vi "外设配置对话框.vi"() -> ()   [LabVIEW 2016, in "斯坦道CODCr.lvlib"]
uses:
  <vilib>/Utility/miscctls.llb/LVPointTypeDef.ctl
panel:
  in  "外设配置":T1 {"总氮x公式0" items=["0", "1"]; "光谱仪类型" items=["1型", "2型", "3型", "2型氙灯联控"]; "泵阀量" items=["9通"=9, "10通"=10, "12通"=12]; "泵类型" items=["1型", "2型", "sy04型+旋转阀"]}
  in  "关闭":bool
  in  "保存":bool
  in  "读取":bool
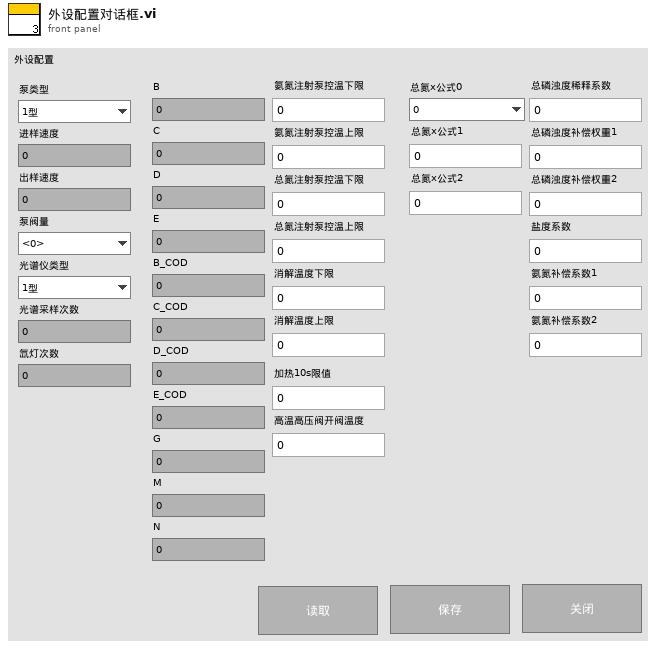
[diagram p1: front panel]
types:
  T1 = cluster{"泵类型":u8, "进样速度":u32, "出样速度":u32, "泵阀量":u8, "光谱仪类型":u8, "光谱采样次数":u8, "氙灯次数":u8, "B":u16, "C":u16, "D":u16, "E":u16, "B_COD":u16, "C_COD":u16, "D_COD":u16, "E_COD":u16, "G":u16, "M":u16, "N":u16, "氨氮注射泵控温下限":sgl, "氨氮注射泵控温上限":sgl, "总氮注射泵控温下限":sgl, "总氮注射泵控温上限":sgl, "消解温度下限":sgl, "消解温度上限":sgl, "加热10s限值":sgl, "高温高压阀开阀温度":sgl, "总氮x公式0":u8, "总氮x公式1":sgl, "总氮x公式2":sgl, "总磷浊度稀释系数":sgl, "总磷浊度补偿权重1":sgl, "总磷浊度补偿权重2":sgl, "盐度系数":sgl, "氨氮补偿系数1":sgl, "氨氮补偿系数2":sgl}
  T2 = typedef "LVPointTypeDef.ctl" = cluster{"Horizontal":i16, "Vertical":i16}
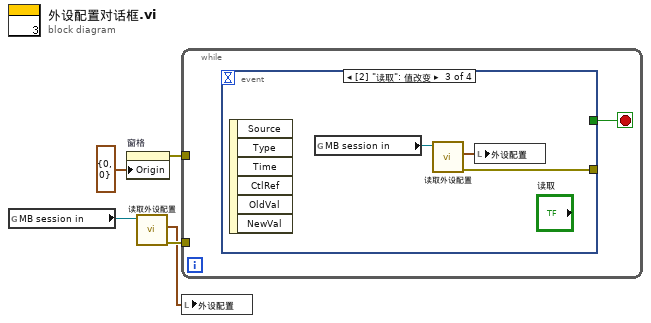
[diagram p0: block diagram]
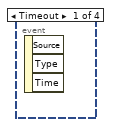
[diagram p2: hidden frame]
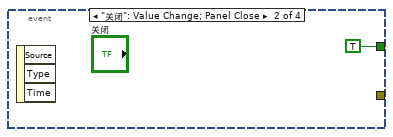
[diagram p3: hidden frame]
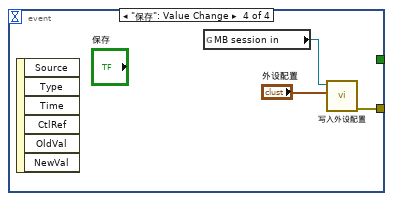
[diagram p4: hidden frame]
diagram:
  n1 = global read "VAR总磷总氮全局变量.vi" "MB session in"() -> (w2:refnum<class "MB_Master.lvclass">)
  n2 = property on="窗格" class="Pane"("Origin"=T2 {"Horizontal"=0, "Vertical"=0} ("原点")) -> (error out=w3:errorcluster)  [unwired: 2 in, 1 out]
  n3 = call "读取外设配置.vi"("MB session in"=w2) -> ("error out"=w5:errorcluster, "外设配置"=w1:T1)  [unwired: 8 in, 1 out]
  n4 = while {
    tunnel: w5 -> [_]
    tunnel: w3 -> [_]
    stop <- w6 stop-if-true
    n5 = event shown="[2] \"读取\": 值改变" {
      selector: _ -> [_ _ _ _]
      dyn-events: _ -> [_ _ _ _]
      timeout: _ -> [_ _ _ _]
      tunnel: [_ TRUE _ _] -> w6
      tunnel: [_ _ w10 w13] -> _
      event Timeout {
        n6 = event-data() -> ()  [unwired: 1 in, 3 out]
      }
      event "关闭": Value Change; Panel Close {
        n7 = event-data() -> ()  [unwired: 1 in, 3 out]
      }
      event "读取": Value Change {
        n8 = event-data() -> ()  [unwired: 1 in, 6 out]
        n9 = global read "VAR总磷总氮全局变量.vi" "MB session in"() -> (w9:refnum<class "MB_Master.lvclass">)
        n10 = call "读取外设配置.vi"("MB session in"=w9) -> ("error out"=w10:errorcluster, "外设配置"=w8:T1)  [unwired: 8 in, 1 out]
        n11 = local write "外设配置"(w8) -> ()
      }
      event "保存": Value Change {
        n12 = event-data() -> ()  [unwired: 1 in, 6 out]
        n13 = global read "VAR总磷总氮全局变量.vi" "MB session in"() -> (w12:refnum<class "MB_Master.lvclass">)
        n14 = call "写入外设配置.vi"("外设配置"="外设配置", "MB session in"=w12) -> ("error out"=w13:errorcluster)  [unwired: 8 in, 1 out]
      }
    }
  }
  n15 = local write "外设配置"(w1) -> ()
